vi "Close.vi"(8 "error in (no error)":errorcluster, 11 "AMS TS3472 in":refnum<class "AMS TCS3472.lvclass">) -> (0 "error out":errorcluster, 3 "AMS TS3472 out":refnum<class "AMS TCS3472.lvclass">)   [LabVIEW 2014, in "AMS TS3472 Light Sensor.lvlib" / "AMS TCS3472.lvclass"]
uses:
  AMS TCS3472.lvclass
  Abstract Sensor/Abstract Sensor.lvclass
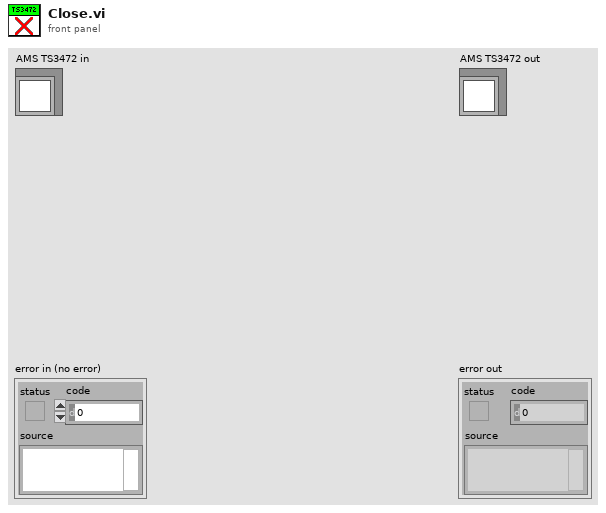
[diagram p1: front panel]
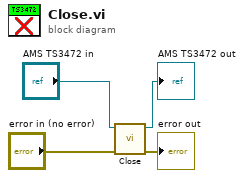
[diagram p0: block diagram]
diagram:
  n1 = call-parent "Close.vi"("error in (no error)"="error in (no error)", "Abstract Sensor in"="AMS TS3472 in") -> ("error out"=→"error out":errorcluster, "Abstract Sensor out"=→"AMS TS3472 out":refnum<class "AMS TCS3472.lvclass">)  [unwired: 8 in]
